vi "Update Shot Table (HIIT).vi"(1 "Sort by AVG":bool, 2 "shot array":T1[](array[typedef]) {"Frag Rod" format="%.1f"; "UncorrectedAvgVel_PB" format="%.1f"; "strikeVel_PB" format="%.1f"; "velLoss_PB" format="%.1f"; "avgVel_PB" format="%.1f"; "Redundant_Velocity" format="%.1f"; "Energy Loss (J)" format="%.3e"; "Projectile Mass" min=0 step=1 format="%.4f"; "Corrected residual" format="%.2f"; "Uncorrected Residual" format="%.2f"; "Corrected Impact" format="%.2f"; "Uncorrected Impact" format="%.2f"; "Shot Angle" max=90 step=1; "SHOT STATUS" items=["Partial", "Complete"]; "IMPACT VELOCITY" min=0 max=10000 step=0.1 format="%.1f"; "Barrel Temperature" format="%.1f"; "Powder Loading" format="%.4f"; "RESIDUAL  VELOCITY" min=0 max=10000 step=0.1 format="%.1f"}) -> (0 "shotTable OUT":string[][](array[string]))   [LabVIEW 2010]
uses:
  Shot Record.ctl
panel:
  in  "HIIT Config":bool=TRUE
  # "Order"
  # "Impact"
  # "Strike Vel"
  # "Residual"
  # "Vel Loss"
  # "Status"
  # "Depth"
  # "Diameter"
  # "Loading"
  # "Description"
  # "Order"
  # "Chrono#1"
  # "Chrono#2"
  # "Average"
  # "Vel Loss"
  # "Strike Vel"
  # "Residual"
  # "Status"
  # "Depth"
  # "Diameter"
  # "Loading"
  # "Description"
  # "Order"
  # "Chrono#1"
  # "Loading"
  # "Status"
  # "Residual"
  # "Depth"
  # "Diameter"
  # "Description"
  # "Chrono#2"
  # "Average"
  # "Vel Loss"
  # "Strike Vel"
  # "Corrected"
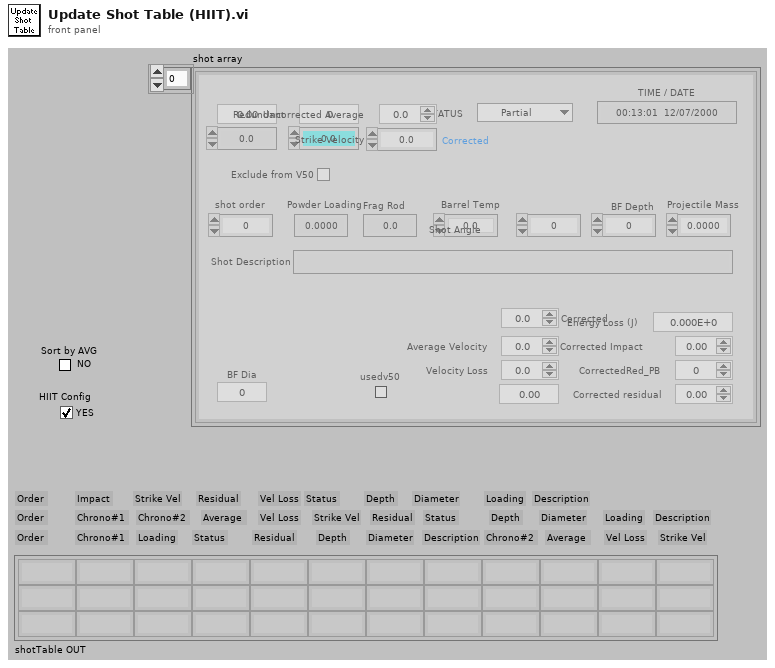
[diagram p1: front panel]
types:
  T1 = typedef "Shot Record.ctl" = cluster{"Uncorrected Impact":sgl, "Uncorrected Residual":sgl, "avgVel_PB":sgl, "IMPACT VELOCITY":sgl, "RESIDUAL  VELOCITY ":sgl, "Shot Description":string, "Powder Loading ":sgl, "Barrel Temperature":sgl, "TIME / DATE":string, "shot order":i32, "SHOT STATUS":u16, "Shot Angle":u16, "Corrected Impact":sgl, "Corrected residual":sgl, "Projectile Mass":sgl, "usedv50":bool, "Energy Loss (J)":sgl, "BackFace\nDepth":sgl, "BackFace\nDiameter":sgl, "Redundant_Velocity":sgl, "velLoss_PB":sgl, "strikeVel_PB":sgl, "UncorrectedRed_PB":sgl, "CorrectedRed_PB":sgl, "UncorrectedAvgVel_PB":sgl, "V50userExcl":bool, "Frag Rod":sgl}
  T2 = cluster{"[0]":string, "[1]":string, "[2]":string, "[3]":string, "[4]":string, "[5]":string, "[6]":string, "[7]":string, "[8]":string, "[9]":string, "[10]":string, "[11]":string}[]
  T3 = cluster{"[0]":string, "[1]":string, "[2]":string, "[3]":string, "[4]":string, "[5]":string, "[6]":string, "[7]":string, "[8]":string, "[9]":string, "[10]":string, "[11]":string}
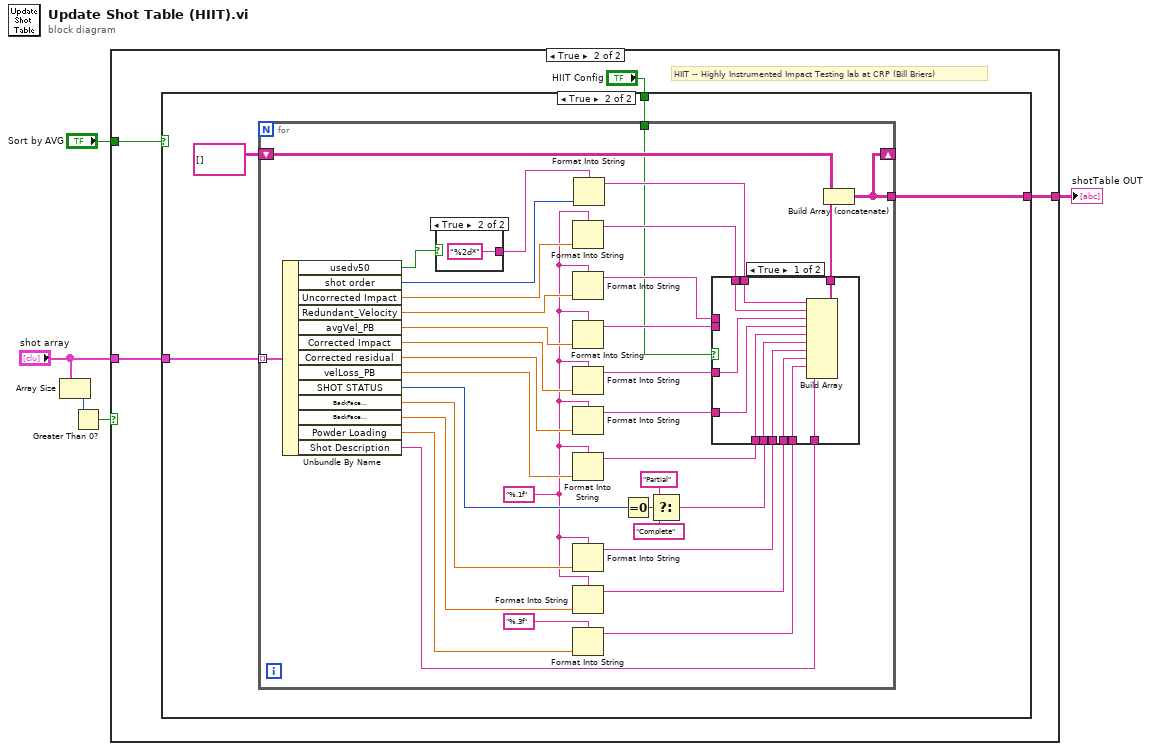
[diagram p0: block diagram]
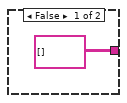
[diagram p2: hidden frame]
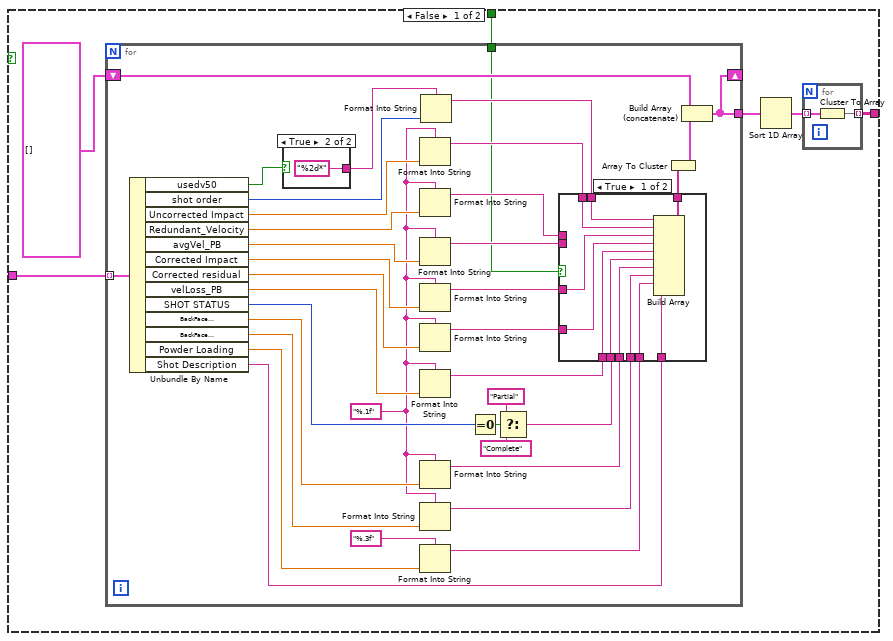
[diagram p3: hidden frame]
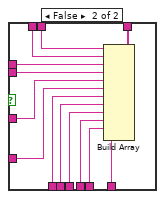
[diagram p4: hidden frame]
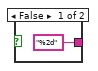
[diagram p5: hidden frame]
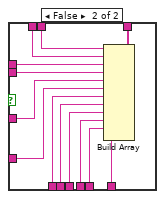
[diagram p6: hidden frame]
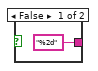
[diagram p7: hidden frame]
diagram:
  n1 = Array Size(array="shot array") -> (size(s)=w5:i32)
  n2 = Greater Than 0?(x=w5) -> (x > 0?=w2:bool)
  n3 = case shown="True" w2 {
    tunnel: "shot array" -> [_ w10]
    tunnel: [string[][] [] w9] -> w3
    tunnel: "Sort by AVG" -> [_ w8]
    frame False {
    }
    frame True {
      # "HIIT -- Highly Instrumented Impact Testing lab at CRP (Bill Briers)"
      n4 = case shown="True" w8 {
        tunnel: w10 -> [w16 w83]
        tunnel: [w14 w82] -> w9
        tunnel: "HIIT Config" -> [w11 w81]
        frame False {
          n5 = for {
            tunnel: w16 -> [w42] mode=indexing
            shift-right: [w50] -> _
            shift-left: T2 [] -> [w54]
            tunnel: [w50] -> w15
            tunnel: w11 -> [w19]
            w21 = "%.1f" ("Format String")
            n6 = Unbundle By Name(w42) -> ("usedv50"=w41:bool, "shot order"=w40:i32, "Uncorrected Impact"=w39:sgl, "Redundant_Velocity"=w38:sgl, "avgVel_PB"=w37:sgl, "Corrected Impact"=w36:sgl, "Corrected residual"=w35:sgl, "velLoss_PB"=w29:sgl, "SHOT STATUS"=w25:u16, "BackFace\nDepth"=w34:sgl, "BackFace\nDiameter"=w33:sgl, "Powder Loading"=w32:sgl, "Shot Description"=w31:string)
            n7 = case shown="True" w41 {
              tunnel: ["%2d" "%2d*"] -> w49
              frame False {
              }
              frame True {
              }
            }
            n8 = Format Into String(format string=w21, w39) -> (resulting string=w51:string)  [unwired: 2 in, 1 out]
            n9 = Format Into String(format string=w21, w38) -> (resulting string=w52:string)  [unwired: 2 in, 1 out]
            n10 = Format Into String(format string=w21, w37) -> (resulting string=w30:string)  [unwired: 2 in, 1 out]
            n11 = Format Into String(format string=w21, w36) -> (resulting string=w47:string)  [unwired: 2 in, 1 out]
            n12 = Format Into String(format string=w21, w35) -> (resulting string=w46:string)  [unwired: 2 in, 1 out]
            n13 = Format Into String(format string=w21, w29) -> (resulting string=w23:string)  [unwired: 2 in, 1 out]
            n14 = Format Into String(format string=w21, w34) -> (resulting string=w45:string)  [unwired: 2 in, 1 out]
            n15 = Format Into String(format string=w21, w33) -> (resulting string=w44:string)  [unwired: 2 in, 1 out]
            n16 = Format Into String(format string="%.3f" ("Format String"), w32) -> (resulting string=w43:string)  [unwired: 2 in, 1 out]
            n17 = Format Into String(format string=w49, w40) -> (resulting string=w48:string)  [unwired: 2 in, 1 out]
            n18 = Equal To 0?(x=w25) -> (x = 0?=w26:bool)
            n19 = Select(t="Partial", s=w26, f="Complete") -> (s? t:f=w24:string)
            n20 = case shown="True" w19 {
              tunnel: [w65 w78] -> w53
              tunnel: w52 -> [_ w77]
              tunnel: w51 -> [w64 w76]
              tunnel: w48 -> [w63 w75]
              tunnel: w47 -> [w62 w74]
              tunnel: w46 -> [w61 w73]
              tunnel: w45 -> [w60 w72]
              tunnel: w44 -> [w59 w71]
              tunnel: w43 -> [w58 w70]
              tunnel: w31 -> [w57 w69]
              tunnel: w30 -> [_ w68]
              tunnel: w24 -> [w56 w67]
              tunnel: w23 -> [w55 w66]
              frame True {
                n21 = Build Array(w63, w64, w62, w61, w55, w56, w60, w59, w58, w57) -> (w65:string[])
              }
              frame False {
                n22 = Build Array(w75, w76, w77, w68, w74, w73, w66, w67, w72, w71, w70, w69) -> (w78:string[])
              }
            }
            n23 = Array To Cluster(array=w53) -> (cluster=w20:T3)
            n24 = Build Array (concatenate)(w54, w20) -> (w50:T2)
          }
          n25 = Sort 1D Array(array=w15) -> (sorted array=w12:T2)
          n26 = for {
            tunnel: w12 -> [w18] mode=indexing
            tunnel: [w17] -> w14 mode=indexing
            n27 = Cluster To Array(cluster=w18) -> (array=w17:string[])
          }
        }
        frame True {
          n28 = for {
            tunnel: w83 -> [w116] mode=indexing
            shift-right: [w118] -> _
            shift-left: string[][] [] -> [w119]
            tunnel: [w118] -> w82
            tunnel: w81 -> [w85]
            w99 = "%.1f" ("Format String")
            n29 = Unbundle By Name(w116) -> ("usedv50"=w115:bool, "shot order"=w114:i32, "Uncorrected Impact"=w113:sgl, "Redundant_Velocity"=w112:sgl, "avgVel_PB"=w111:sgl, "Corrected Impact"=w110:sgl, "Corrected residual"=w109:sgl, "velLoss_PB"=w105:sgl, "SHOT STATUS"=w101:u16, "BackFace\nDepth"=w108:sgl, "BackFace\nDiameter"=w107:sgl, "Powder Loading"=w106:sgl, "Shot Description"=w98:string)
            n30 = case shown="True" w115 {
              tunnel: ["%2d" "%2d*"] -> w117
              frame False {
              }
              frame True {
              }
            }
            n31 = Format Into String(format string=w99, w113) -> (resulting string=w88:string)  [unwired: 2 in, 1 out]
            n32 = Format Into String(format string=w99, w112) -> (resulting string=w86:string)  [unwired: 2 in, 1 out]
            n33 = Format Into String(format string=w99, w111) -> (resulting string=w87:string)  [unwired: 2 in, 1 out]
            n34 = Format Into String(format string=w99, w110) -> (resulting string=w91:string)  [unwired: 2 in, 1 out]
            n35 = Format Into String(format string=w99, w109) -> (resulting string=w92:string)  [unwired: 2 in, 1 out]
            n36 = Format Into String(format string=w99, w105) -> (resulting string=w93:string)  [unwired: 2 in, 1 out]
            n37 = Format Into String(format string=w99, w108) -> (resulting string=w95:string)  [unwired: 2 in, 1 out]
            n38 = Format Into String(format string=w99, w107) -> (resulting string=w96:string)  [unwired: 2 in, 1 out]
            n39 = Format Into String(format string="%.3f" ("Format String"), w106) -> (resulting string=w97:string)  [unwired: 2 in, 1 out]
            n40 = Format Into String(format string=w117, w114) -> (resulting string=w89:string)  [unwired: 2 in, 1 out]
            n41 = Equal To 0?(x=w101) -> (x = 0?=w102:bool)
            n42 = Select(t="Partial", s=w102, f="Complete") -> (s? t:f=w94:string)
            n43 = case shown="True" w85 {
              tunnel: [w130 w143] -> w90
              tunnel: w86 -> [_ w142]
              tunnel: w88 -> [w129 w141]
              tunnel: w89 -> [w128 w140]
              tunnel: w91 -> [w127 w139]
              tunnel: w92 -> [w126 w138]
              tunnel: w95 -> [w125 w137]
              tunnel: w96 -> [w124 w136]
              tunnel: w97 -> [w123 w135]
              tunnel: w98 -> [w122 w134]
              tunnel: w87 -> [_ w133]
              tunnel: w94 -> [w121 w132]
              tunnel: w93 -> [w120 w131]
              frame True {
                n44 = Build Array(w128, w129, w127, w126, w120, w121, w125, w124, w123, w122) -> (w130:string[])
              }
              frame False {
                n45 = Build Array(w140, w141, w142, w133, w139, w138, w131, w132, w137, w136, w135, w134) -> (w143:string[])
              }
            }
            n46 = Build Array (concatenate)(w119, w90) -> (w118:string[][])
          }
        }
      }
    }
  }
  "shotTable OUT" <- w3
